vi "MDAQ_AnalysisProgram.vi"() -> ()   [LabVIEW 2021]
uses:
  FunctionVIS/ANAL_State.ctl
  FunctionVIS/ANAL_Data.ctl
  FunctionVIS/XML_Cluster.ctl
  FunctionVIS/DAT_Cluster.ctl
  FunctionVIS/ANAL_GUIStatus.ctl
  446bc6b8-02c6-443f-b214-55262fd3fba4.vi
  446bc6b8-02c6-443f-b214-55262fd3fba4.vi/d4db2432-cc9c-482c-8957-dac855435ef6.vi
  446bc6b8-02c6-443f-b214-55262fd3fba4.vi/86fbf154-bd7b-49a2-8ab2-a837b2a95f24.vi
  446bc6b8-02c6-443f-b214-55262fd3fba4.vi/3b95b01e-1ec2-4565-bcd9-7606a5281010.vi
  446bc6b8-02c6-443f-b214-55262fd3fba4.vi/96a08935-737a-44b2-979c-a81d56408f7e.vi
  446bc6b8-02c6-443f-b214-55262fd3fba4.vi/d4db2432-cc9c-482c-8957-dac855435ef6.vi/6eaecd13-6e48-4772-a921-b51ebdf84d88.vi
  446bc6b8-02c6-443f-b214-55262fd3fba4.vi/d4db2432-cc9c-482c-8957-dac855435ef6.vi/d2d5f2b7-06f4-47f6-971c-049c3fdbb653.vi
  446bc6b8-02c6-443f-b214-55262fd3fba4.vi/3b95b01e-1ec2-4565-bcd9-7606a5281010.vi/6eaecd13-6e48-4772-a921-b51ebdf84d88.vi
  446bc6b8-02c6-443f-b214-55262fd3fba4.vi/3b95b01e-1ec2-4565-bcd9-7606a5281010.vi/d2d5f2b7-06f4-47f6-971c-049c3fdbb653.vi
  446bc6b8-02c6-443f-b214-55262fd3fba4.vi/96a08935-737a-44b2-979c-a81d56408f7e.vi/6eaecd13-6e48-4772-a921-b51ebdf84d88.vi
  446bc6b8-02c6-443f-b214-55262fd3fba4.vi/96a08935-737a-44b2-979c-a81d56408f7e.vi/d2d5f2b7-06f4-47f6-971c-049c3fdbb653.vi
  <vilib>/Comparison/Less/Less Functor/Less Functor.lvclass
panel:
  out "Tics":i32
  in  "Exit_Button":bool
  in  "Tab Control":enum32{"Data Overview", "Data Visualisation"}(tab)
  in  "LoadOld_Button":bool
  out "Amplitude Range":string
  out "Temperature Range":string
  in  "Source File Tree":string[](tree)
  in  "Remove_Button":bool
  in  "Prev_Button":bool
  in  "Next_Button":bool
  out "ID":u32
  out "Aprox Delta T (s)":dbl
  out "Run End Time":timestamp format="%<%x %X>T"
  out "No. Scans":u32
  out "No. SetPoints":u32
  out "Target Bins/Ampl":i32[](array[numeric])
  out "User Comments":string
  out "Sample Name":string
  out "Run Start Time":timestamp format="%<%x %X>T"
  in  "Load_Button":bool
  in  "Temperature":bool
  in  "Normalise to Sweep Number?":bool
  in  "Software Gate":cluster{"Numeric":i32, "Numeric":i32}(slide)={"Numeric"=96, "Numeric"=937} scale=0.0..1023.0
  in  "Refresh_Button":bool
  in  "Scan Range":cluster{"Numeric":i32, "Numeric":i32}(slide)={"Numeric"=1, "Numeric"=58} scale=1.0..12.0
  in  "Tab Control 2":T1(tab)
  in  "Delete_Button":bool
  in  "Bin/Amplitude":i32(slide) scale=0.0..6000.0
  out "Waveform Graph":i32[](graph)
  out "Time Plot":T2(graph)
  out "Temperature Plot":T3(graph)
  out "Amp Plot":cluster{"Numeric":i32, dbl}[](graph)
  out "Intensity Graph":dbl[][](graph)
  in  "Scan Selection":i32(slide)=1 min=1 max=58 step=1 scale=1.0..12.0
  # "Selected Master File Info:"
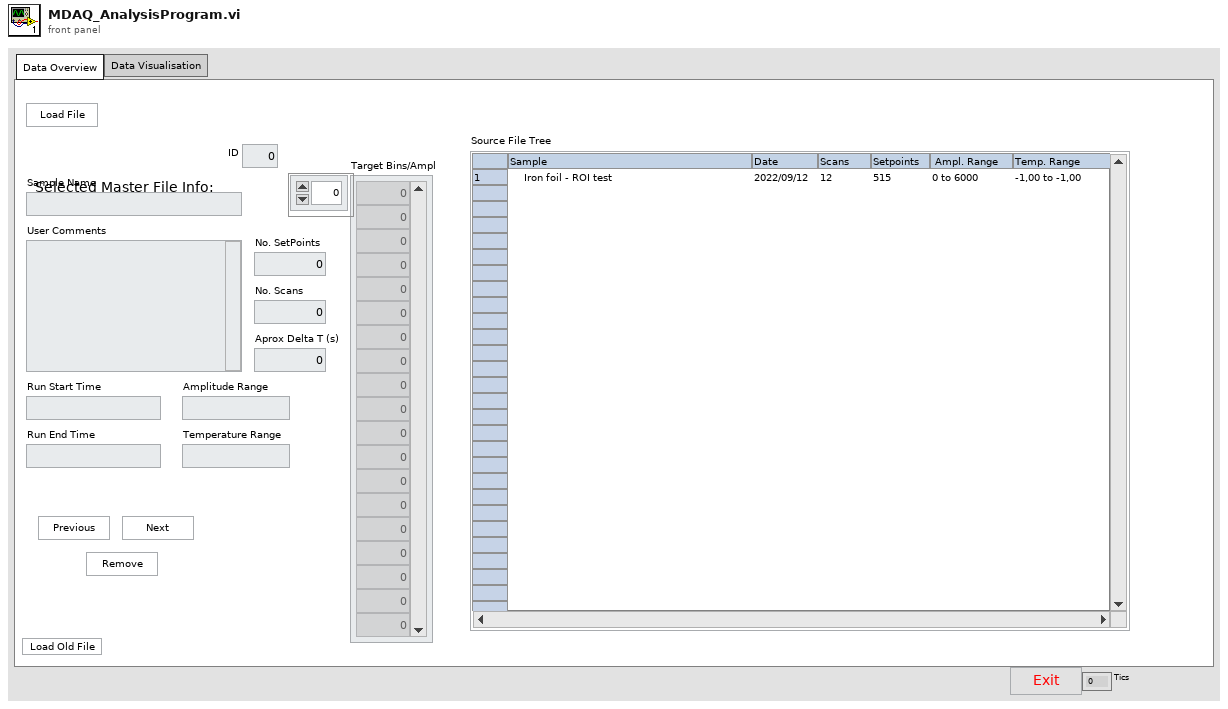
[diagram p1: front panel]
types:
  T1 = enum32{"Spectrum Reviewer", "Time Plot", "Temperature Plot", "Amplitude Plot", "Surface Review"}
  T2 = cluster{"Counts Array":cluster{timestamp, dbl}[]}[]
  T3 = cluster{"Counts Array":cluster{"Avg Temp":dbl, i32}[]}[]
  T4 = typedef "ANAL_GUIStatus.ctl" = cluster{"Display Index":i32, "Number Of Files":u32, "Last Added ID":u32}
  T5 = typedef "ANAL_Data.ctl" = cluster{"Run Info Out":T6, "Run Data Cluster":T7, "ID":u32, "Derived Data":cluster{"No. Cycles":u32, "Aprox Delta":dbl, "Run End Time":timestamp, "Ampl Range":string, "Temp Range":string}}[]
  T6 = typedef "XML_Cluster.ctl" = cluster{"User Comment":string, "Run Start TimeS":timestamp, "No. Set Points":u32, "Target Set Points":i32[], "Sample Name":string}
  T7 = typedef "DAT_Cluster.ctl" = cluster{"Bin Start Time":timestamp, "Temperature A":dbl, "Temperature B":dbl, "Sweep No.":i32, "Bin Value":i32, "Raw MDAQ Counts":i32[]}[]
  T8 = typedef "ANAL_State.ctl" = enum16{"DeleteSingleSpectrum", "RefreshSpectPlot", "RefreshPlotUI", "RefreshPlots", "UpdateTree", "DeriveData", "RemItem", "PrevItem", "NextItem", "Refresh", "LoadOldFile", "Load File", "Idle", "ProgInit"}
  T9 = cluster{"Run Info Out":T6, "Run Data Cluster":T7, "ID":u32, "Derived Data":cluster{"No. Cycles":u32, "Aprox Delta":dbl, "Run End Time":timestamp, "Ampl Range":string, "Temp Range":string}}
  T10 = cluster{"No. Cycles":u32, "Aprox Delta":dbl, "Run End Time":timestamp, "Ampl Range":string, "Temp Range":string}
  T11 = typedef "ANAL_TREECluster.ctl" = cluster{"IDs":string[], "Sample Names":string[], "Start Times":string[], "Sweeps":string[], "Set Points":string[], "Amp Ranges":string[], "Temp Ranges":string[]}
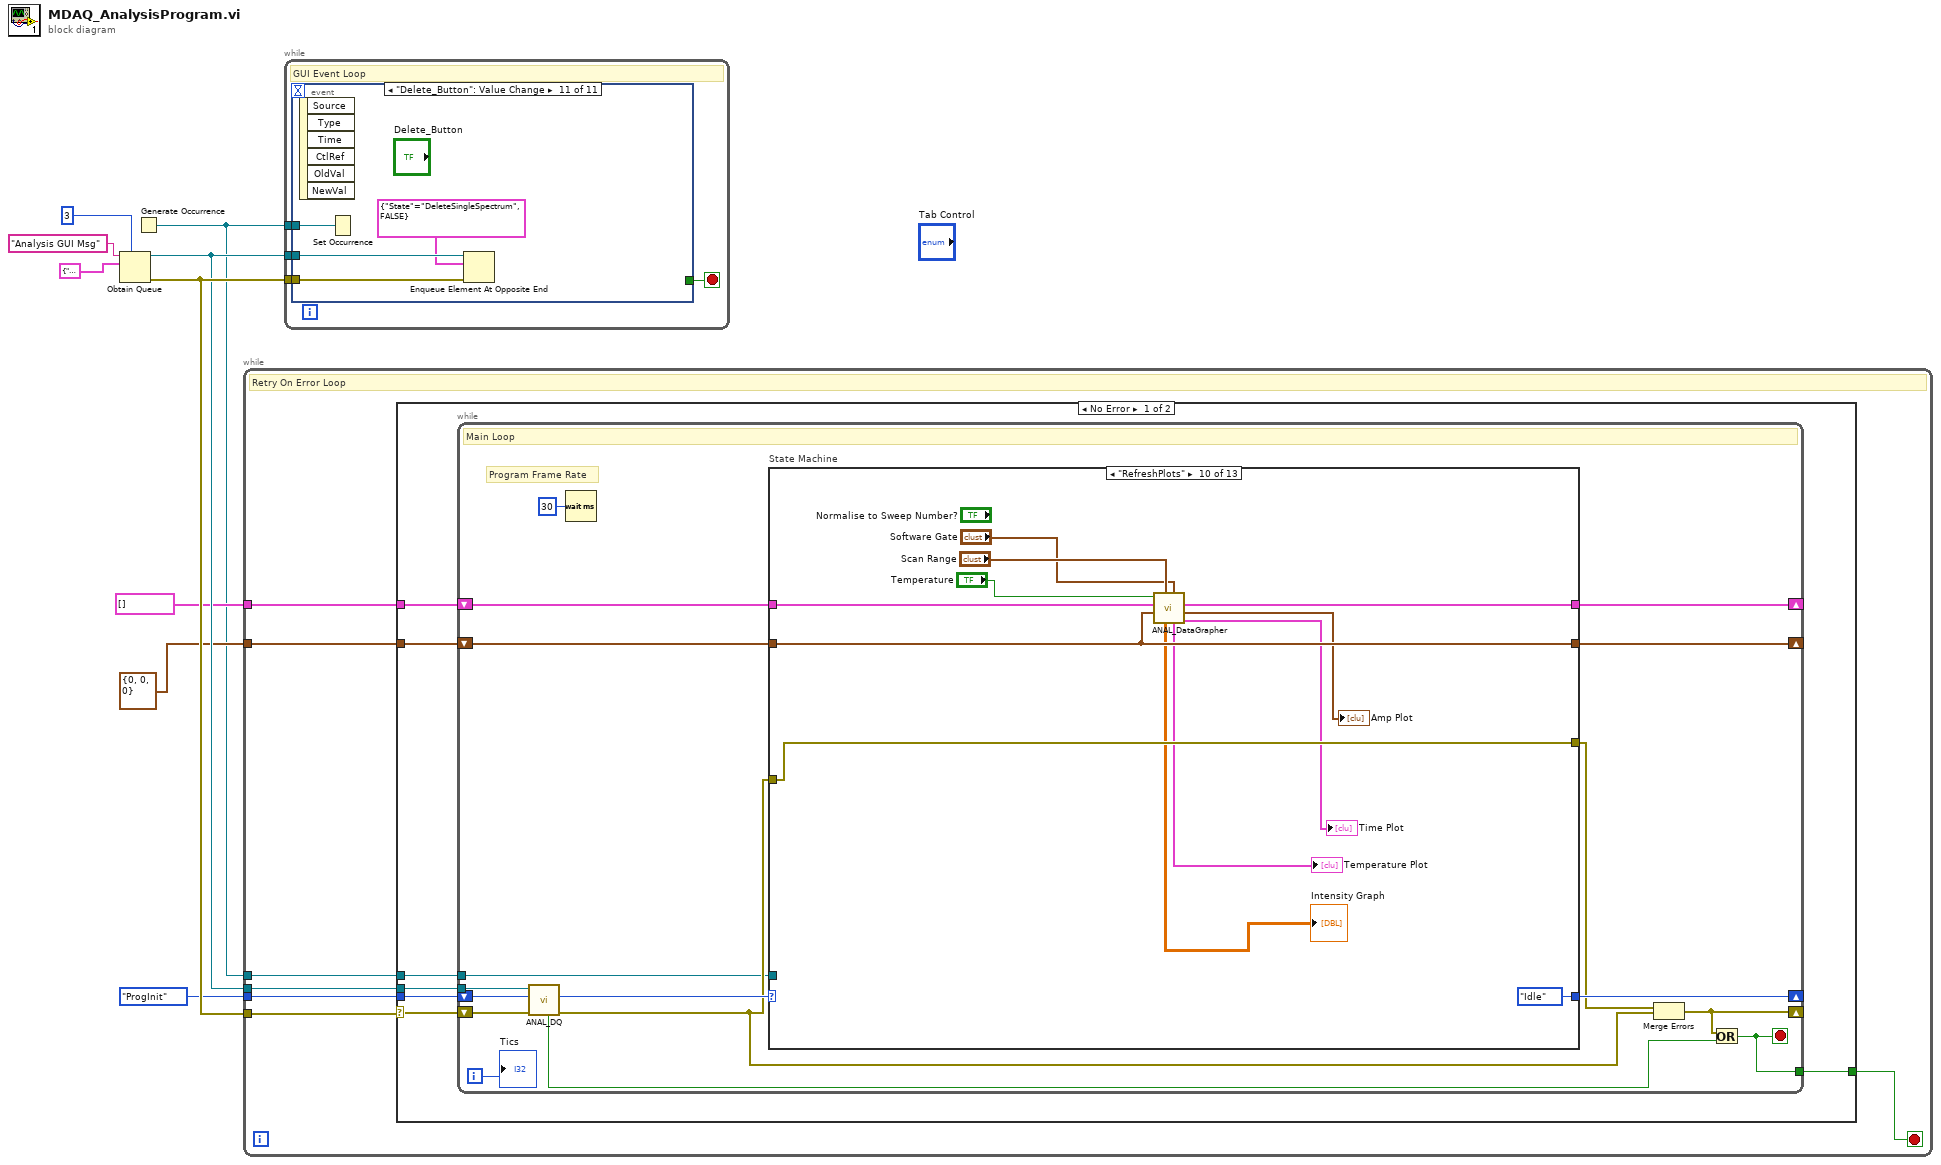
[diagram p0: block diagram]
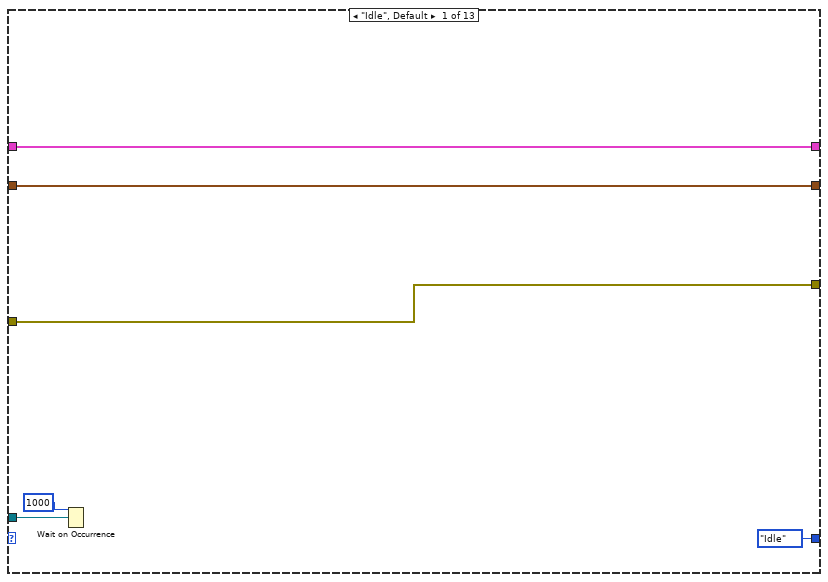
[diagram p2: hidden frame]
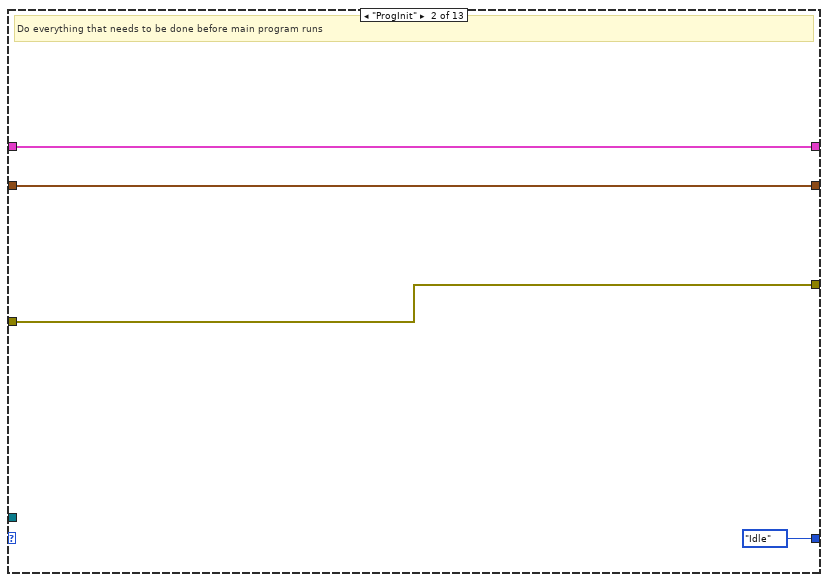
[diagram p3: hidden frame]
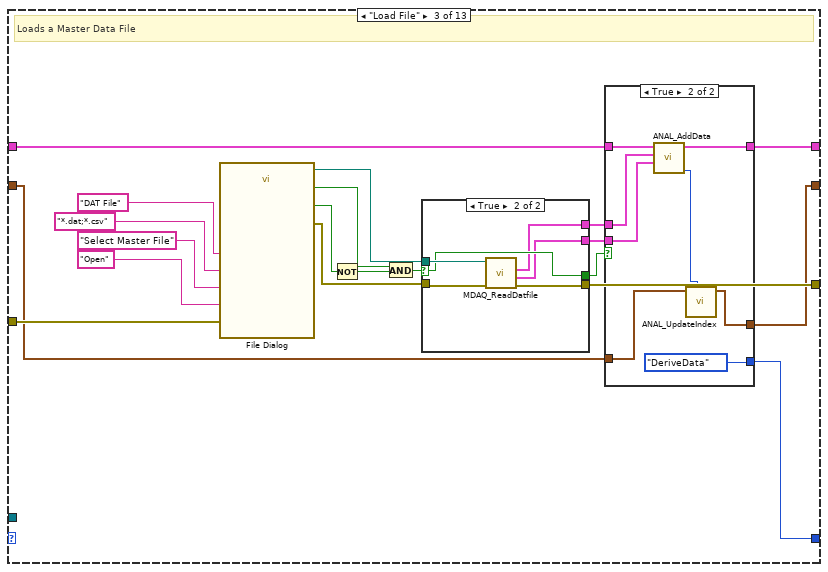
[diagram p4: hidden frame]
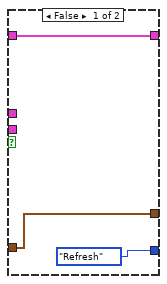
[diagram p5: hidden frame]
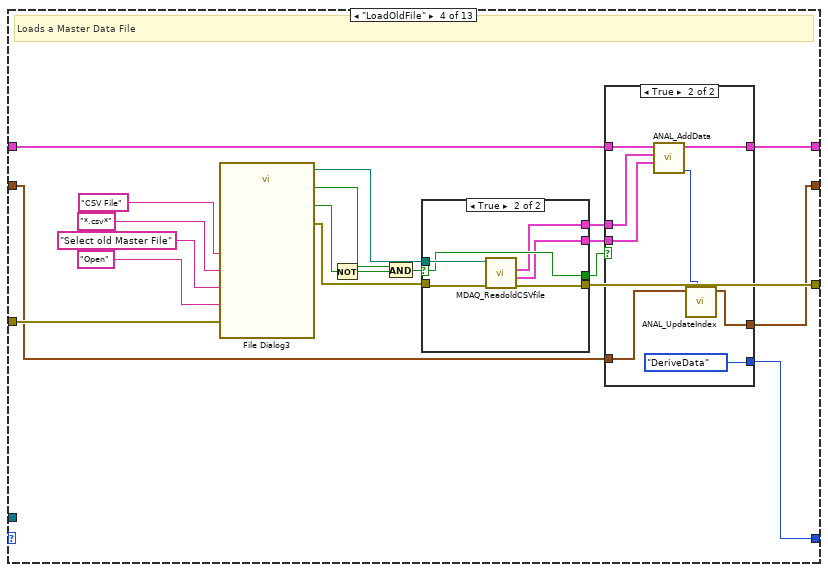
[diagram p7: hidden frame]
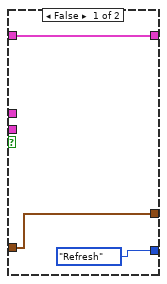
[diagram p8: hidden frame]
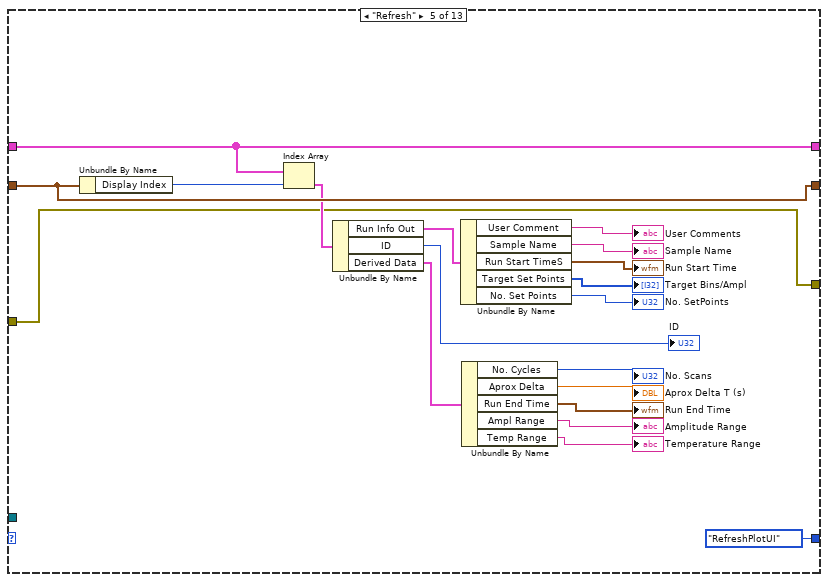
[diagram p10: hidden frame]
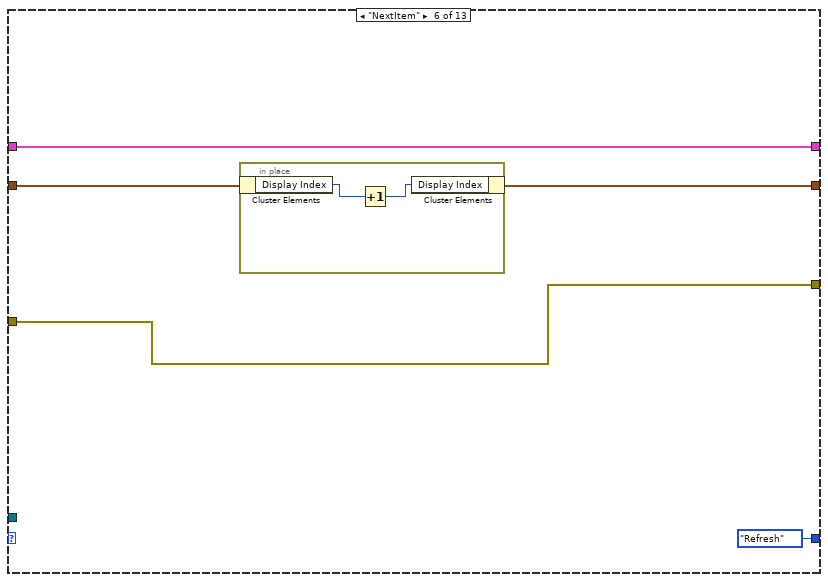
[diagram p11: hidden frame]
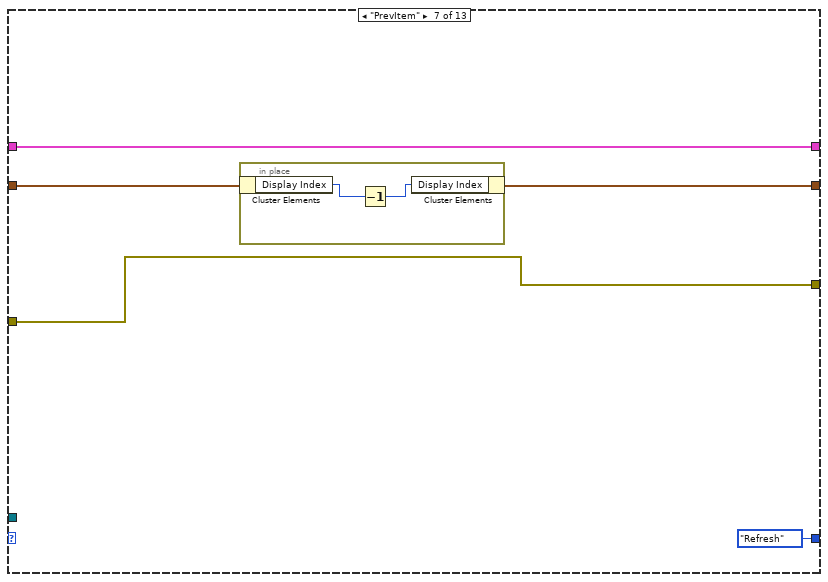
[diagram p12: hidden frame]
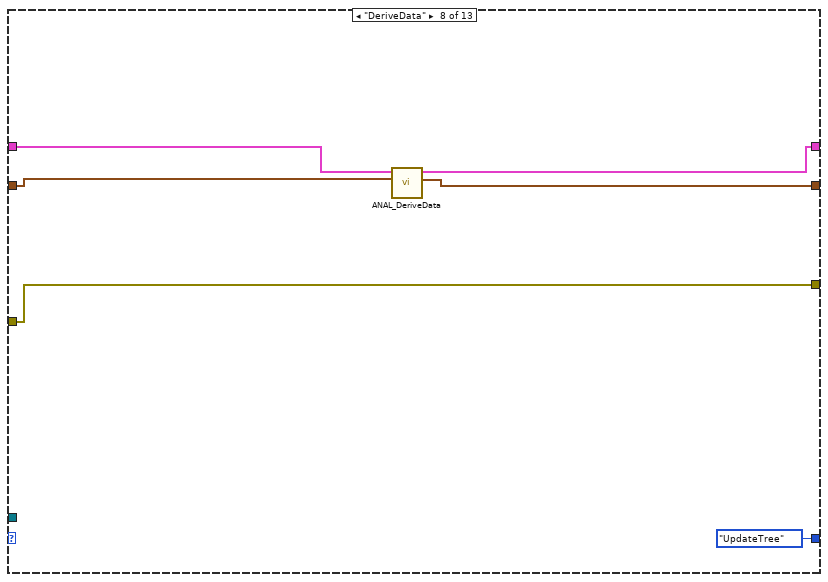
[diagram p13: hidden frame]
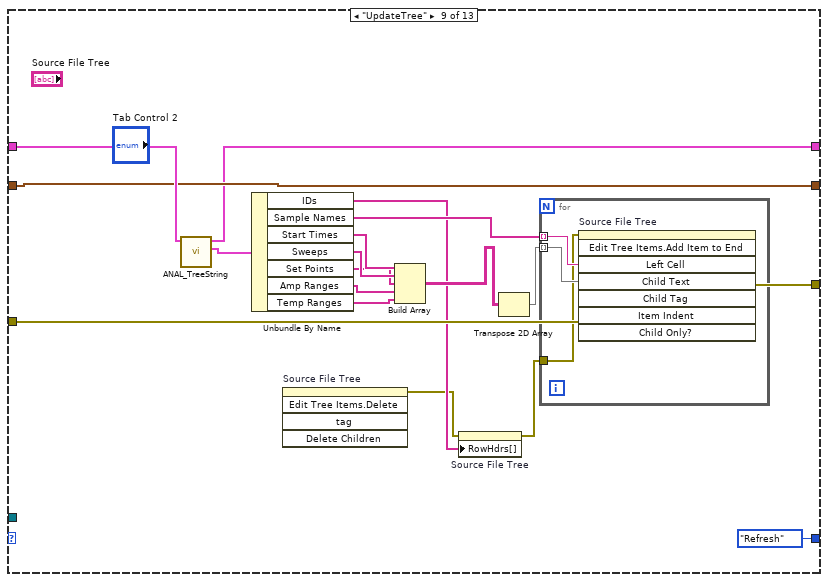
[diagram p14: hidden frame]
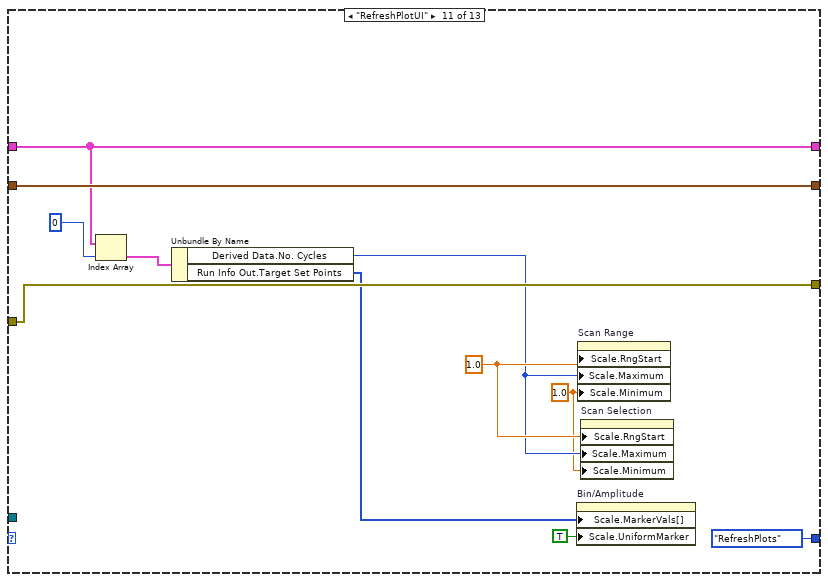
[diagram p15: hidden frame]
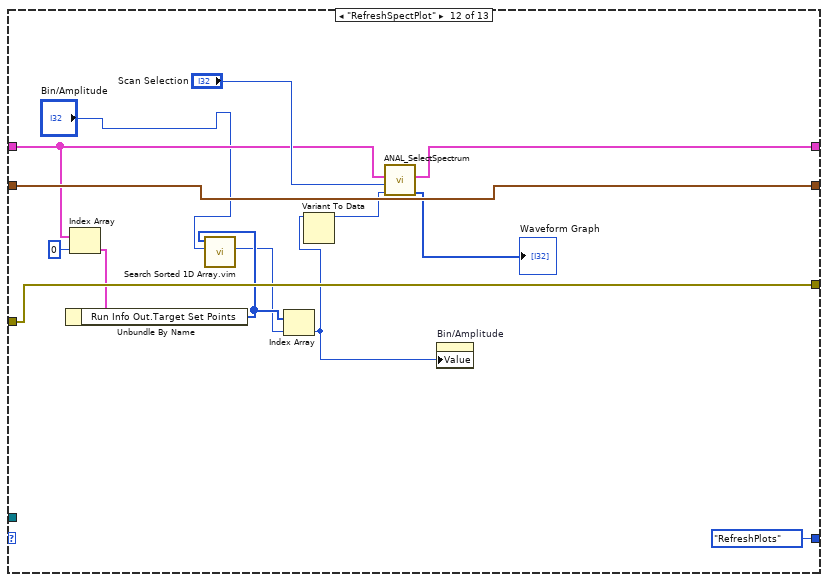
[diagram p16: hidden frame]
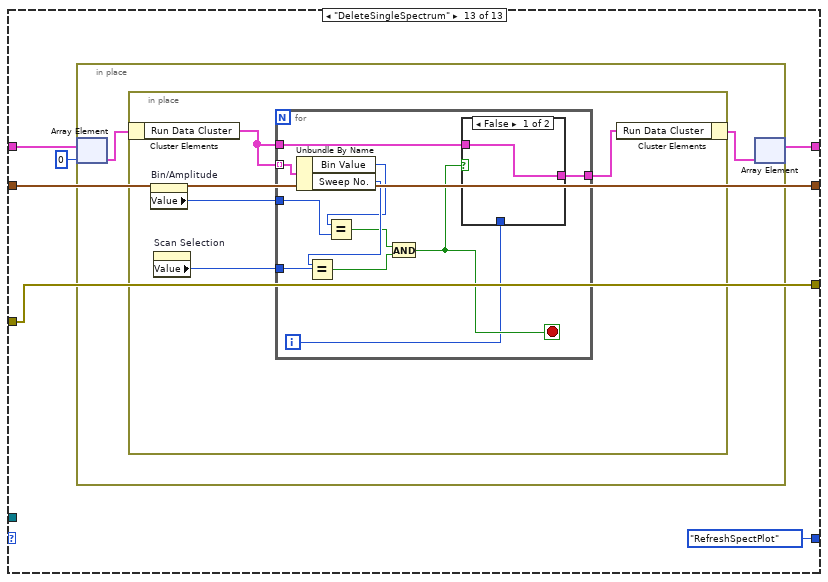
[diagram p17: hidden frame]
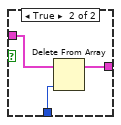
[diagram p18: hidden frame]
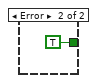
[diagram p19: hidden frame]
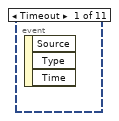
[diagram p20: hidden frame]
diagram:
  n1 = Obtain Queue(max queue size (-1, unlimited)=3, name (unnamed)="Analysis GUI Msg", element data type=cluster{"State":T8, bool} {"State"=enum."ProgInit", TRUE}) -> (queue out=w5:refnum<queue>, error out=w6:errorcluster)  [unwired: 2 in, 1 out]
  n2 = Generate Occurrence() -> (w1:refnum<k4>)
  n3 = while {
    tunnel: w6 -> [w16]
    tunnel: w5 -> [w15]
    tunnel: ANAL_State."ProgInit" ("State") -> [w14]
    tunnel: T5 [] ("Main Data Array") -> [w12]
    tunnel: T4 {"Display Index"=0, "Number Of Files"=0, "Last Added ID"=0} ("GUI Cluster") -> [w11]
    tunnel: w1 -> [w10]
    stop <- w13 stop-if-true
    # "Retry On Error Loop"
    n4 = case shown="No Error" w16 {
      selector: w16 -> [w23 _]
      tunnel: w15 -> [w22 _]
      tunnel: w14 -> [w21 _]
      tunnel: [w20 TRUE] -> w13
      tunnel: w12 -> [w19 _]
      tunnel: w11 -> [w18 _]
      tunnel: w10 -> [w17 _]
      frame No Error {
        n5 = while {
          tunnel: w22 -> [w33]
          shift-right: [w34] -> _
          shift-left: w21 -> [w39]
          tunnel: [w36] -> w20
          shift-right: [w28] -> _
          shift-left: w19 -> [w35]
          shift-right: [w29] -> _
          shift-left: w23 -> [w31]
          shift-right: [w26] -> _
          shift-left: w18 -> [w27]
          tunnel: w17 -> [w25]
          i -> [w24]
          stop <- w36 stop-if-true
          # "Program Frame Rate"
          # "Main Loop"
          n6 = call "ANAL_DQ.vi"("error in (no error)"=w31, "State"=w39, "queue In"=w33) -> ("error out"=w30:errorcluster, "State Out"=w38:T8, "Exit?"=w37:bool)  [unwired: 6 in]
          n7 = Wait (ms)(milliseconds to wait=u32 30) -> ()  [unwired: 1 out]
          n8 = case "State Machine" shown="\"RefreshPlots\"" w38 {
            tunnel: w35 -> [w46 w49 w58 w97 w147 w152 w159 w167 w184 w197 w207 w217 w227]
            tunnel: [ANAL_State."Idle" ("State") ANAL_State."Idle" ("State") w53 w92 ANAL_State."RefreshPlotUI" ("State") ANAL_State."Refresh" ("State") ANAL_State."Refresh" ("State") ANAL_State."UpdateTree" ("State") ANAL_State."Refresh" ("State") ANAL_State."Idle" ("State") ANAL_State."RefreshPlots" ("State") ANAL_State."RefreshPlots" ("State") ANAL_State."RefreshSpectPlot" ("State")] -> w34
            tunnel: w30 -> [w44 w47 w66 w105 w138 w151 w158 w163 w182 w199 w209 w222 w229]
            tunnel: [w44 w47 w59 w98 w138 w151 w158 w163 w182 w199 w209 w222 w229] -> w32
            tunnel: [w46 w49 w54 w93 w147 w152 w159 w166 w179 w196 w207 w224 w225] -> w28
            tunnel: w27 -> [w45 w48 w52 w91 w146 w149 w156 w165 w183 w195 w210 w223 w230]
            tunnel: [w45 w48 w51 w90 w146 w148 w155 w164 w183 w195 w210 w223 w230] -> w26
            tunnel: w25 -> [w42 _ _ _ _ _ _ _ _ _ _ _ _]
            frame "Idle", Default {
              n9 = Wait on Occurrence(2:w42, 3:1000 ("ms timeout (-1)")) -> ()  [unwired: 1 in, 1 out]
            }
            frame "ProgInit" {
              # "Do everything that needs to be done before main program runs"
            }
            frame "Load File" {
              # "Loads a Master Data File"
              n10 = call "File Dialog"("prompt"="Select Master File", "button label"="Open", "error in"=w66, "pattern (all files)"="*.dat;*.csv", "pattern label"="DAT File") -> ("selected path"=w60:path, "exists"=w63:bool, "cancelled"=w61:bool, "error out"=w65:errorcluster)  [unwired: 7 in]
              n11 = Not(x=w61) -> (.not. x?=w62:bool)
              n12 = And(x=w63, y=w62) -> (x .and. y?=w64:bool)
              n13 = case shown="True" w64 {
                selector: w64 -> [w82 w86]
                tunnel: w65 -> [w83 w89]
                tunnel: w60 -> [_ w88]
                tunnel: [w83 w87] -> w59
                tunnel: [w82 w86] -> w57
                tunnel: [_ w85] -> w56
                tunnel: [_ w84] -> w55
                frame False {
                }
                frame True {
                  n14 = call "MDAQ_ReadDatfile.vi"("error in"=w89, "file path (use dialog)"=w88) -> ("error out"=w87:errorcluster, "Run Data Cluster"=w84:T7, "Run Info Out"=w85:T6)  [unwired: 7 in]
                }
              }
              n15 = case shown="True" w57 {
                tunnel: w58 -> [w73 w81]
                tunnel: w56 -> [_ w80]
                tunnel: w55 -> [_ w79]
                tunnel: [w73 w78] -> w54
                tunnel: [ANAL_State."Refresh" ("State") ANAL_State."DeriveData" ("State")] -> w53
                tunnel: w52 -> [w71 w76]
                tunnel: [w71 w75] -> w51
                frame False {
                }
                frame True {
                  n16 = call "ANAL_AddData.vi"("Run Data Cluster In"=w79, "Run Info In"=w80, "Main Data Array"=w81) -> ("ID"=w74:u32, "output array"=w78:T5)  [unwired: 7 in]
                  n17 = call "ANAL_UpdateIndex.vi"("ID Added"=w74, "GUI Cluster in"=w76) -> ("GUI Cluster out"=w75:T4)  [unwired: 9 in]
                }
              }
            }
            frame "LoadOldFile" {
              # "Loads a Master Data File"
              n18 = call "File Dialog3"("prompt"="Select old Master File", "button label"="Open", "error in"=w105, "pattern (all files)"="*.csv*", "pattern label"="CSV File") -> ("selected path"=w99:path, "exists"=w102:bool, "cancelled"=w100:bool, "error out"=w104:errorcluster)  [unwired: 7 in]
              n19 = Not(x=w100) -> (.not. x?=w101:bool)
              n20 = And(x=w102, y=w101) -> (x .and. y?=w103:bool)
              n21 = case shown="True" w103 {
                selector: w103 -> [w121 w125]
                tunnel: w104 -> [w122 w128]
                tunnel: w99 -> [_ w127]
                tunnel: [w122 w126] -> w98
                tunnel: [w121 w125] -> w96
                tunnel: [_ w124] -> w95
                tunnel: [_ w123] -> w94
                frame False {
                }
                frame True {
                  n22 = call "MDAQ_ReadoldCSVfile.vi"("error in"=w128, "file path (use dialog)"=w127) -> ("error out"=w126:errorcluster, "Run Data Cluster"=w123:T7, "Run Info Out"=w124:T6)  [unwired: 7 in]
                }
              }
              n23 = case shown="True" w96 {
                tunnel: w97 -> [w112 w120]
                tunnel: w95 -> [_ w119]
                tunnel: w94 -> [_ w118]
                tunnel: [w112 w117] -> w93
                tunnel: [ANAL_State."Refresh" ("State") ANAL_State."DeriveData" ("State")] -> w92
                tunnel: w91 -> [w110 w115]
                tunnel: [w110 w114] -> w90
                frame False {
                }
                frame True {
                  n24 = call "ANAL_AddData.vi"("Run Data Cluster In"=w118, "Run Info In"=w119, "Main Data Array"=w120) -> ("ID"=w113:u32, "output array"=w117:T5)  [unwired: 7 in]
                  n25 = call "ANAL_UpdateIndex.vi"("ID Added"=w113, "GUI Cluster in"=w115) -> ("GUI Cluster out"=w114:T4)  [unwired: 9 in]
                }
              }
            }
            frame "Refresh" {
              n26 = Unbundle By Name(w146) -> ("Display Index"=w135:i32)
              n27 = Index Array(array=w147, index=w135) -> (element=w145:T9)
              n28 = Unbundle By Name(w145) -> ("Run Info Out"=w144:T6, "ID"=→"ID":u32, "Derived Data"=w134:T10)
              n29 = Unbundle By Name(w144) -> ("User Comment"=→"User Comments":string, "Sample Name"=→"Sample Name":string, "Run Start TimeS"=→"Run Start Time":timestamp, "Target Set Points"=→"Target Bins/Ampl":i32[], "No. Set Points"=→"No. SetPoints":u32)
              n30 = Unbundle By Name(w134) -> ("No. Cycles"=→"No. Scans":u32, "Aprox Delta"=→"Aprox Delta T (s)":dbl, "Run End Time"=→"Run End Time":timestamp, "Ampl Range"=→"Amplitude Range":string, "Temp Range"=→"Temperature Range":string)
            }
            frame "NextItem" {
              n31 = in-place {
                n32 = in-place-cluster #1(w149) -> ("Display Index"=w154:i32)
                n33 = Increment(x=w154) -> (x+1=w153:i32)
                n34 = in-place-cluster #1("Display Index"=w153) -> (w148:T4)
              }
            }
            frame "PrevItem" {
              n35 = in-place {
                n36 = in-place-cluster #2(w156) -> ("Display Index"=w161:i32)
                n37 = Decrement(x=w161) -> (x-1=w160:i32)
                n38 = in-place-cluster #2("Display Index"=w160) -> (w155:T4)
              }
            }
            frame "DeriveData" {
              n39 = call "ANAL_DeriveData.vi"("GUI Cluster"=w165, "Main Data Array"=w167) -> ("GUI Cluster Out"=w164:T4, "Main Data Array Out"=w166:T5)  [unwired: 8 in]
            }
            frame "UpdateTree" {
              n40 = call "ANAL_TreeString.vi"("Main Data Array"=w184) -> ("Tree Cluster Out"=w180:T11, "Main Data Array 2"=w179:T5)  [unwired: 9 in]
              n41 = Unbundle By Name(w180) -> ("IDs"=w170:string[], "Sample Names"=w173:string[], "Start Times"=w178:string[], "Sweeps"=w177:string[], "Set Points"=w176:string[], "Amp Ranges"=w175:string[], "Temp Ranges"=w174:string[])
              n42 = invoke on="Source File Tree" class="Tree (strict)" method="Edit Tree Items.Delete"() -> (error out=w169:errorcluster)  [unwired: 5 in, 4 out]
              n43 = Build Array(w178, w177, w176, w175, w174) -> (w172:string[][])
              n44 = property on="Source File Tree" class="Tree (strict)"(error in=w169, "RowHdrs[]"=w170) -> (error out=w168:errorcluster)  [unwired: 1 in, 1 out]
              n45 = Transpose 2D Array(2D array=w172) -> (transposed array=w171:string[][])
              n46 = for {
                tunnel: w171 -> [w187] mode=indexing
                tunnel: w173 -> [w186] mode=indexing
                tunnel: w168 -> [w185]
                n47 = invoke on="Source File Tree" class="Tree (strict)" method="Edit Tree Items.Add Item to End"(error in=w185, "Left Cell"=w186, "Child Text"=w187) -> ()  [unwired: 5 in, 8 out]
              }
            }
            frame "RefreshPlots" {
              n48 = call "ANAL_DataGrapher.vi"("Software Gate"="Software Gate", "Sweep Range"="Scan Range", "GUI Cluster"=w195, "Main Data Array"=w197, "AorB"="Temperature") -> ("Time Array"=→"Time Plot":T2, "Bin Graph"=→"Amp Plot":cluster{"Numeric":i32, dbl}[], "Main Data Array Out"=w196:T5, "Temp Array"=→"Temperature Plot":T3, "Normalised Surface"=→"Intensity Graph":dbl[][])  [unwired: 2 in]
            }
            frame "RefreshPlotUI" {
              w202 = 1.0 ("Scale.Range:Minimum")
              w204 = 1.0 ("Scale.Range:Start")
              n49 = Index Array(array=w207, index=0) -> (element=w205:T9)
              n50 = Unbundle By Name(w205) -> ("Derived Data.No. Cycles"=w203:u32, "Run Info Out.Target Set Points"=w201:i32[])
              n51 = property on="Bin/Amplitude" class="Slide (strict)"("Scale.MarkerVals[]"=w201, "Scale.UniformMarker"=TRUE ("Scale.Uniform Marker Spacing?")) -> ()  [unwired: 2 in, 2 out]
              n52 = property on="Scan Range" class="Slide (strict)"("Scale.RngStart"=w204, "Scale.Maximum"=w203, "Scale.Minimum"=w202) -> ()  [unwired: 2 in, 2 out]
              n53 = property on="Scan Selection" class="Slide (strict)"("Scale.RngStart"=w204, "Scale.Maximum"=w203, "Scale.Minimum"=w202) -> ()  [unwired: 2 in, 2 out]
            }
            frame "RefreshSpectPlot" {
              n54 = Index Array(array=w217, index=0) -> (element=w215:T9)
              n55 = Unbundle By Name(w215) -> ("Run Info Out.Target Set Points"=w213:i32[])
              n56 = call "Search Sorted 1D Array.vim"("element"="Bin/Amplitude", "sorted 1D array"=w213) -> ("nearest index"=w212:i32)  [unwired: 8 in, 1 out]
              n57 = Index Array(array=w213, index=w212) -> (element=w211:i32)
              n58 = Variant To Data(Variant=w211) -> (data=w218:i32)  [unwired: 2 in, 1 out]
              n59 = call "ANAL_SelectSpectrum.vi"("Single Bin Selection"=w218, "Sweep Selection"="Scan Selection", "Main Data Array"=w217) -> ("Selected Spectrum"=→"Waveform Graph":i32[], "Main Data Array Out"=w224:T5)  [unwired: 7 in]
              n60 = property on="Bin/Amplitude" class="Slide (strict)"("Value"=w211) -> ()  [unwired: 2 in, 2 out]
            }
            frame "DeleteSingleSpectrum" {
              n61 = in-place {
                n62 = in-place-array #3(w227, 0) -> (w232:T9)
                n63 = in-place {
                  n64 = in-place-cluster #4(w232) -> ("Run Data Cluster"=w234:T7)
                  n65 = property on="Bin/Amplitude" class="Slide (strict)"() -> ("Value"=w236:i32)  [unwired: 2 in, 2 out]
                  n66 = property on="Scan Selection" class="Slide (strict)"() -> ("Value"=w235:i32)  [unwired: 2 in, 2 out]
                  n67 = for {
                    tunnel: w234 -> [w247] mode=indexing
                    tunnel: w236 -> [w244]
                    tunnel: w235 -> [w246]
                    tunnel: w234 -> [w240]
                    tunnel: [w237] -> w233
                    i -> [w238]
                    stop <- w239 stop-if-true
                    n68 = Unbundle By Name(w247) -> ("Bin Value"=w243:i32, "Sweep No."=w245:i32)
                    n69 = Equal?(x=w245, y=w246) -> (x = y?=w241:bool)
                    n70 = Equal?(x=w243, y=w244) -> (x = y?=w242:bool)
                    n71 = And(x=w242, y=w241) -> (x .and. y?=w239:bool)
                    n72 = case shown="False" w239 {
                      tunnel: w240 -> [w248 w251]
                      tunnel: w238 -> [_ w250]
                      tunnel: [w248 w249] -> w237
                      frame False {
                      }
                      frame True {
                        n73 = Delete From Array(array=w251, index=w250) -> (array with subset deleted=w249:T7)  [unwired: 1 in, 1 out]
                      }
                    }
                  }
                  n74 = in-place-cluster #4("Run Data Cluster"=w233) -> (w231:T9)
                }
                n75 = in-place-array #3(w231) -> (w225:T5)  [unwired: 1 out]
              }
            }
          }
          n76 = Merge Errors(w32, w30) -> (w29:errorcluster)
          n77 = Or(x=w29, y=w37) -> (x .or. y?=w36:bool)
          "Tics" <- w24
        }
      }
      frame Error {
      }
    }
  }
  n78 = while {
    tunnel: w5 -> [w256]
    tunnel: w6 -> [w255]
    tunnel: w1 -> [w253]
    stop <- w254 stop-if-true
    # "GUI Event Loop"
    n79 = event shown="[10] \"Delete_Button\": Value Change" {
      selector: _ -> [_ _ _ _ _ _ _ _ _ _ _]
      dyn-events: _ -> [_ _ _ _ _ _ _ _ _ _ _]
      timeout: _ -> [_ _ _ _ _ _ _ _ _ _ _]
      tunnel: w256 -> [_ w261 w265 w269 w273 w277 w281 w285 w289 w293 w297]
      tunnel: w255 -> [_ w260 w264 w268 w272 w276 w280 w284 w288 w292 w296]
      tunnel: [_ TRUE _ _ _ _ _ _ _ _ _] -> w254
      tunnel: w253 -> [_ w257 w262 w266 w270 w274 w278 w282 w286 w290 w294]
      event Timeout {
        n80 = event-data() -> ()  [unwired: 1 in, 3 out]
      }
      event "Exit_Button": Value Change {
        n81 = event-data() -> ()  [unwired: 1 in, 6 out]
        n82 = Set Occurrence(w257) -> ()
        n83 = Enqueue Element At Opposite End(queue=w261, element=cluster{"State":T8, bool} {"State"=enum."Idle", TRUE}, error in (no error)=w260) -> ()  [unwired: 1 in, 3 out]
      }
      event "Load_Button": Value Change {
        n84 = event-data() -> ()  [unwired: 1 in, 6 out]
        n85 = Set Occurrence(w262) -> ()
        n86 = Enqueue Element At Opposite End(queue=w265, element=cluster{"State":T8, bool} {"State"=enum."Load File", FALSE}, error in (no error)=w264) -> ()  [unwired: 1 in, 3 out]
      }
      event "LoadOld_Button": Value Change {
        n87 = event-data() -> ()  [unwired: 1 in, 6 out]
        n88 = Set Occurrence(w266) -> ()
        n89 = Enqueue Element At Opposite End(queue=w269, element=cluster{"State":T8, bool} {"State"=enum."LoadOldFile", FALSE}, error in (no error)=w268) -> ()  [unwired: 1 in, 3 out]
      }
      event "Next_Button": Value Change {
        n90 = event-data() -> ()  [unwired: 1 in, 6 out]
        n91 = Set Occurrence(w270) -> ()
        n92 = Enqueue Element At Opposite End(queue=w273, element=cluster{"State":T8, bool} {"State"=enum."NextItem", FALSE}, error in (no error)=w272) -> ()  [unwired: 1 in, 3 out]
      }
      event "Prev_Button": Value Change {
        n93 = event-data() -> ()  [unwired: 1 in, 6 out]
        n94 = Set Occurrence(w274) -> ()
        n95 = Enqueue Element At Opposite End(queue=w277, element=cluster{"State":T8, bool} {"State"=enum."PrevItem", FALSE}, error in (no error)=w276) -> ()  [unwired: 1 in, 3 out]
      }
      event "Remove_Button": Value Change {
        n96 = event-data() -> ()  [unwired: 1 in, 6 out]
        n97 = Set Occurrence(w278) -> ()
        n98 = Enqueue Element At Opposite End(queue=w281, element=cluster{"State":T8, bool} {"State"=enum."RemItem", FALSE}, error in (no error)=w280) -> ()  [unwired: 1 in, 3 out]
      }
      event "Refresh_Button": Value Change {
        n99 = event-data() -> ()  [unwired: 1 in, 6 out]
        n100 = Set Occurrence(w282) -> ()
        n101 = Enqueue Element At Opposite End(queue=w285, element=cluster{"State":T8, bool} {"State"=enum."RefreshPlots", FALSE}, error in (no error)=w284) -> ()  [unwired: 1 in, 3 out]
      }
      event "Software Gate", "Scan Range": Value Change {
        n102 = event-data() -> ()  [unwired: 1 in, 6 out]
        n103 = Set Occurrence(w286) -> ()
        n104 = Enqueue Element At Opposite End(queue=w289, element=cluster{"State":T8, bool} {"State"=enum."RefreshPlots", FALSE}, error in (no error)=w288) -> ()  [unwired: 1 in, 3 out]
      }
      event "Scan Selection", "Bin/Amplitude": Value Change {
        n105 = event-data() -> ()  [unwired: 1 in, 6 out]
        n106 = Set Occurrence(w290) -> ()
        n107 = Enqueue Element At Opposite End(queue=w293, element=cluster{"State":T8, bool} {"State"=enum."RefreshSpectPlot", FALSE}, error in (no error)=w292) -> ()  [unwired: 1 in, 3 out]
      }
      event "Delete_Button": Value Change {
        n108 = event-data() -> ()  [unwired: 1 in, 6 out]
        n109 = Set Occurrence(w294) -> ()
        n110 = Enqueue Element At Opposite End(queue=w297, element=cluster{"State":T8, bool} {"State"=enum."DeleteSingleSpectrum", FALSE}, error in (no error)=w296) -> ()  [unwired: 1 in, 3 out]
      }
    }
  }
